vi "Style Tests - Heading 2 Style.vi"(8 "error in (no error)":errorcluster) -> (0 "error out":errorcluster)   [LabVIEW 2020]
uses:
  src/Styles/Underline--ring.ctl
  src/Styles/Alignment--ring.ctl
  src/Styles/Heading 2/Heading 2.lvclass
  D:/Benjamin/Documents/Perso/Code/WC/LabVIEW_NPOI/src/Styles/Style/Style.lvclass
  src/Styles/Style/Get Color (Hex).vi
  src/Styles/Style/Get Style Name.vi
  <vilib>/addons/_JKI Toolkits/Caraya/classes/Assert/Assert Equal Value and Type_Variant.vi
  <vilib>/addons/_JKI Toolkits/Caraya/classes/Assert/Assert False.vi
  <vilib>/addons/_JKI Toolkits/Caraya/classes/Assert/Assert Equal Value_Variant.vi
  <vilib>/addons/_JKI Toolkits/Caraya/classes/Test/Test.lvclass
  <vilib>/addons/_JKI Toolkits/Caraya/classes/Assert/Assert.lvclass
  src/Styles/Styles.lvlib
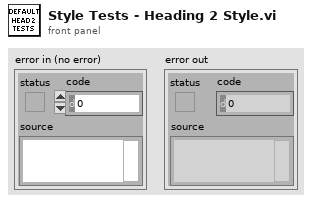
[diagram p1: front panel]
types:
  T1 = typedef "Styles.lvlib/Alignment--ring.ctl" = i32
  T2 = typedef "Styles.lvlib/Underline--ring.ctl" = i32
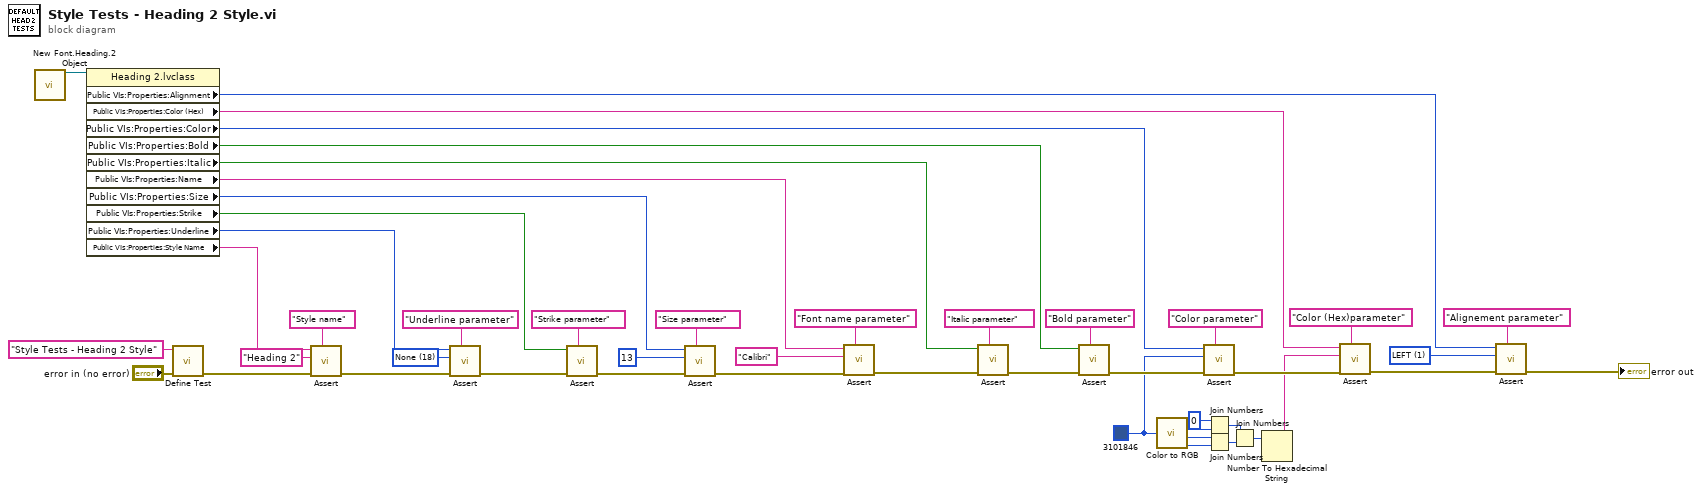
[diagram p0: block diagram]
diagram:
  w6 = T1 1 items=["LEFT"=1, "CENTER"=2, "RIGHT"=3, "BOTH"=4, "MEDIUM_KASHIDA"=5, "DISTRIBUTE"=6, "NUM_TAB"=7, "HIGH_KASHIDA"=8, "LOW_KASHIDA"=9, "THAI_DISTRIBUTE"=10] ("Style:Alignment")
  w15 = u32 3101846 ("Color")
  w37 = T2 18 items=["Single"=1, "Words"=2, "Double"=3, "Thick"=4, "Dotted"=5, "DottedHeavy"=6, "Dash"=7, "DashedHeavy"=8, "DashLong"=9, "DashLongHeavy"=10, "DotDash"=11, "DashDotHeavy"=12, "DotDotDash"=13, "DashDotDotHeavy"=14, "Wave"=15, "WavyHeavy"=16, "WavyDouble"=17, "None"=18] ("Style:Underline")
  n1 = call "New Font.Heading.2 Object.vi"() -> ("Heading 2 out"=w39:refnum<class "Heading 2.lvclass">)  [unwired: 10 in, 1 out]
  n2 = property class="Heading 2.lvclass"(reference=w39) -> ("Public VIs:Properties:Alignment"=w7:T1, "Public VIs:Properties:Color (Hex)"=w12:string, "Public VIs:Properties:Color"=w16:u32, "Public VIs:Properties:Bold"=w26:bool, "Public VIs:Properties:Italic"=w30:bool, "Public VIs:Properties:Name"=w33:string, "Public VIs:Properties:Size"=w35:i32, "Public VIs:Properties:Strike"=w36:bool, "Public VIs:Properties:Underline"=w38:T2, "Public VIs:Properties:Style Name"=w2:string)  [unwired: 1 in, 2 out]
  n3 = call <vilib>:"Define Test.vi"("error in (no error)"="error in (no error)", "Label (VI Title)"="Style Tests - Heading 2 Style") -> ("error out"=w5:errorcluster)  [unwired: 9 in]
  n4 = call-poly <vilib>:"Assert.vi"("Label"="Style name", "error in (no error)"=w5, "Y"="Heading 2" ("Label"), "X"=w2) -> ("error out"=w4:errorcluster)  [unwired: 7 in]
  n5 = call-poly <vilib>:"Assert.vi"("Label"="Underline parameter", "error in (no error)"=w4, "Y"=w37, "X"=w38) -> ("error out"=w47:errorcluster)  [unwired: 7 in]
  n6 = call-poly <vilib>:"Assert.vi"("Label"="Strike parameter", "error in (no error)"=w47, "False?"=w36) -> ("error out"=w42:errorcluster)  [unwired: 8 in]
  n7 = call-poly <vilib>:"Assert.vi"("Label"="Size parameter", "error in (no error)"=w42, "Y"=13 ("Style:Size"), "X"=w35) -> ("error out"=w41:errorcluster)  [unwired: 7 in]
  n8 = call-poly <vilib>:"Assert.vi"("Label"="Font name parameter", "error in (no error)"=w41, "Y"="Calibri" ("Label"), "X"=w33) -> ("error out"=w29:errorcluster)  [unwired: 7 in]
  n9 = call-poly <vilib>:"Assert.vi"("Label"="Italic parameter", "error in (no error)"=w29, "False?"=w30) -> ("error out"=w27:errorcluster)  [unwired: 8 in]
  n10 = call-poly <vilib>:"Assert.vi"("Label"="Bold parameter", "error in (no error)"=w27, "False?"=w26) -> ("error out"=w17:errorcluster)  [unwired: 8 in]
  n11 = call <vilib>:"Color to RGB.vi"("Color"=w15) -> ("R"=w25:u8, "G"=w24:u8, "B"=w23:u8)  [unwired: 1 out]
  n12 = call-poly <vilib>:"Assert.vi"("Label"="Color parameter", "error in (no error)"=w17, "Y"=w15, "X"=w16) -> ("error out"=w13:errorcluster)  [unwired: 7 in]
  n13 = Join Numbers(hi=u8 0, lo=w25) -> ((hi.lo)=w21:u16)
  n14 = Join Numbers(hi=w24, lo=w23) -> ((hi.lo)=w20:u16)
  n15 = Join Numbers(hi=w21, lo=w20) -> ((hi.lo)=w19:u32)
  n16 = Number To Hexadecimal String(2:w19) -> (0:w11:string)  [unwired: 1 in]
  n17 = call-poly <vilib>:"Assert.vi"("Label"="Color (Hex)parameter", "error in (no error)"=w13, "Y"=w11, "X"=w12) -> ("error out"=w9:errorcluster)  [unwired: 7 in]
  n18 = call-poly <vilib>:"Assert.vi"("Label"="Alignement parameter", "error in (no error)"=w9, "Y"=w6, "X"=w7) -> ("error out"=→"error out":errorcluster)  [unwired: 7 in]
